vi "ATS_SetExtRegClock.vi"(8 "rate":enum16{"500M", "250M", "125M"}(ring), 10 "Clock":T1 {"ClckEdge" items=["Rising", "Falling"]; "ClckRate" items=["1 kS/s", "2 kS/s", "5 kS/s", "10 kS/s", "20 kS/s", "50 kS/s", "100 kS/s", "200 kS/s", "500 kS/s", "1 MS/s", "2 MS/s", "5 MS/s", "10 MS/s", "20 MS/s", "25 MS/s", "50 MS/s", "100 MS/s", "200 MS/s", "500 MS/s", "1 GS/s"]}, 11 "DeviceIn":i32) -> (0 "Return Code":u32, 3 "DeviceOut":i32)   [LabVIEW 2017]
doc: "_____AlazarTech, Scope_____\n\nConfigure the capture clock circuitry."
uses:
  AlazarTech/ATS-VI/6.3.0/ATS_ctl/Clock.ctl
  AlazarTech/ATS-VI/6.3.0/ATS_ctl/ClockSource.ctl
  AlazarTech/ATS-VI/6.3.0/ATS_ctl/ClockRate.ctl
  AlazarTech/ATS-VI/6.3.0/ATS_ctl/ClockEdge.ctl
  AlazarTech/ATS-VI/6.3.0/ATS_ctl/ATS_Global_Ctrl.ctl
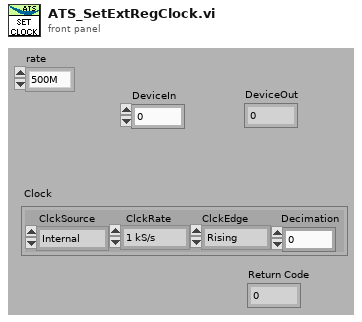
[diagram p1: front panel]
types:
  T1 = typedef "Clock.ctl" = cluster{"ClckSource":T2, "ClckRate":T3, "ClckEdge":T4, "Decimation":u32}
  T2 = typedef "ClockSource.ctl" = enum16{"Internal", "External", "Medium Ext.", "Slow Ext.", "Ext. AC", "Ext. DC", "Ext. (PLL)"}
  T3 = typedef "ClockRate.ctl" = u32
  T4 = typedef "ClockEdge.ctl" = u16
  T5 = typedef "ATS_Global_Ctrl.ctl" = enum16{"Init_Device", "Clear_ALL", "Set", "Get"}
  T6 = typedef "ATS_Set_Value.ctl" = cluster{"Clock (s)":dbl, "RangeA (v)":dbl, "RangeB (v)":dbl, "Ranges (v)":dbl[]}
  T7 = typedef "ATS_Global_4Ch.ctl" = cluster{"Record":T8, "Clock":T1, "Inputs":T9, "Trigger":T15}
  T8 = typedef "Record.ctl" = cluster{"Count":u32, "Presize":u32, "Length":u32}
  T9 = typedef "ATS_InputArray.ctl" = T10[]
  T10 = typedef "InputCtrl.ctl" = cluster{"Coupling":T11, "Range":T12, "Impedance":T13, "Bandwidth":T14}
  T11 = typedef "Coupling.ctl" = enum16{"AC", "DC"}
  T12 = typedef "Range.ctl" = u32
  T13 = typedef "Impedance.ctl" = enum16{"1M ohms", "50 ohms"}
  T14 = typedef "Bandwidth.ctl" = enum16{"Full Bandwidth", "Reduce Bandwidth"}
  T15 = typedef "ATS_Trigger_4Ch.ctl" = cluster{"TrigOperation":T16, "Timeout (s)":dbl, "Trig. Delay":u32, "Engine X":T17, "Engine Y":T17, "ExtTrigControl":T19}
  T16 = typedef "TriggerOperation.ctl" = enum16{"Only X", "Only Y", "X or Y", "X and Y", "X xor Y", "X and not Y", "not X and Y"}
  T17 = typedef "ATS_TriggerEngine_4Ch.ctl" = cluster{"Source":T18, "Slope":enum32{"Positive", "Negative"}, "Level":u32}
  T18 = typedef "ATS_TriggerSource_4Ch.ctl" = enum32{"Chan_A", "Chan_B", "External", "Disable", "Chan_C", "Chan_D"}
  T19 = typedef "ExtTrigger.ctl" = cluster{"Coupling":T11, "Range":T20}
  T20 = typedef "ExtTrigRange.ctl" = enum16{"1 V", "5 V", "TTL", "2.5 V"}
  T21 = typedef "Device_Info.ctl" = cluster{"Handle":u32, "Board":string, "CPLD":string, "MemorySize":u32, "SampleSize":u8, "ID":i32, "High_Memory":bool, "Chan/Board":u8}
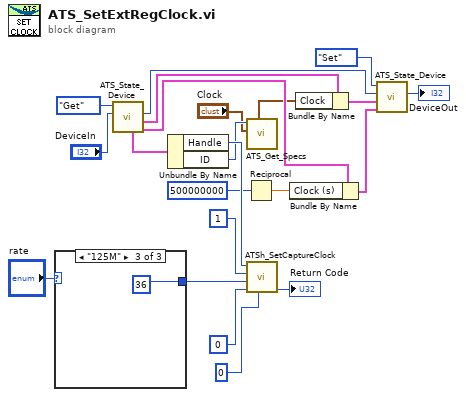
[diagram p0: block diagram]
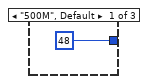
[diagram p2: hidden frame]
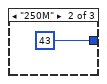
[diagram p3: hidden frame]
diagram:
  n1 = case shown="\"125M\"" "rate" {
    tunnel: [u32 48 ("Rate") u32 43 ("Rate") u32 36 ("Rate")] -> w2
    frame "500M", Default {
    }
    frame "250M" {
    }
    frame "125M" {
    }
  }
  n2 = call "ATS_State_Device.vi"("DeviceIn"="DeviceIn", "ATS_GBL_Ctrl"=ATS_Global_Ctrl."Get") -> ("Ref_Out"=w14:T6, "SetupOut"=w15:T7, "DeviceOut"=w19:i32, "DevInfo_Out"=w13:T21)  [unwired: 4 in, 2 out]
  n3 = Unbundle By Name(w13) -> ("Handle"=w17:u32, "ID"=w11:i32)
  n4 = Reciprocal(x=u32 500000000 ("Rate")) -> (1/x=w5:dbl)
  n5 = call "ATS_Get_Specs.vi"("Clock_Input"="Clock", "ID"=w11) -> ("Clock_Output"=w9:T1)  [unwired: 1 in, 8 out]
  n6 = call "ATSh_SetCaptureClock.vi"("Decimation"=u32 0, "Edge"=u32 0 ("Operation"), "Rate"=w2, "Source"=u32 1 ("Operation"), "Handle"=w17) -> ("Return"=→"Return Code":u32)  [unwired: 6 out]
  n7 = Bundle By Name(cluster=w14, "Clock (s)"=w5) -> (w12:T6)
  n8 = Bundle By Name(cluster=w15, "Clock"=w9) -> (w16:T7)
  n9 = call "ATS_State_Device.vi"("Ref_In"=w12, "SetupIn"=w16, "DeviceIn"=w19, "ATS_GBL_Ctrl"=ATS_Global_Ctrl."Set") -> ("DeviceOut"=→"DeviceOut":i32)  [unwired: 2 in, 5 out]
